vi "Read Interactive.vi"(11 "Test Runner in":refnum<class "Test Runner.lvclass">) -> (2 "Interactive":bool, 3 "Test Runner out":refnum<class "Test Runner.lvclass">)   [LabVIEW 2013, in "Caraya.lvlib" / "Test Runner.lvclass"]
uses:
  Test Runner.lvclass
  Test Runner.lvclass/Test Runner.ctl
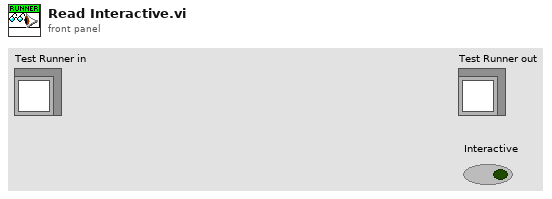
[diagram p1: front panel]
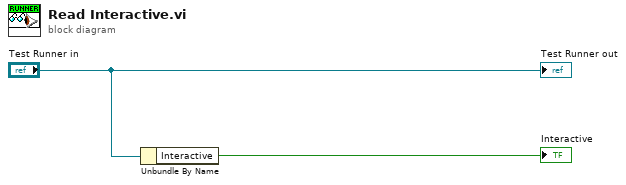
[diagram p0: block diagram]
diagram:
  n1 = Unbundle By Name("Test Runner in") -> ("Interactive"=→"Interactive":bool)
  "Test Runner out" <- "Test Runner in"
